vi "_script_uid_display.vi"(9 "Show uid? (F)":bool, 10 "uids":string[](array[string]), 11 "defaults":cluster{"uid":string, "name":string}[](array[cluster])) -> (3 "display":string[](array[string]))   [LabVIEW 2019, in "Script.lvlib"]
doc: "Displays the shortcut with or without the unique identifier formatted as <short name> | <vi>:<arg>.\n\nExample: \"Connect Pane | support\\Builtins.vi:c\"\n\nCreated by: Ryan Pacini"
uses:
  Script.lvlib
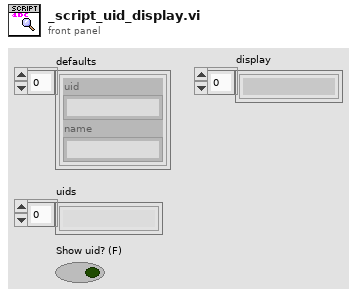
[diagram p1: front panel]
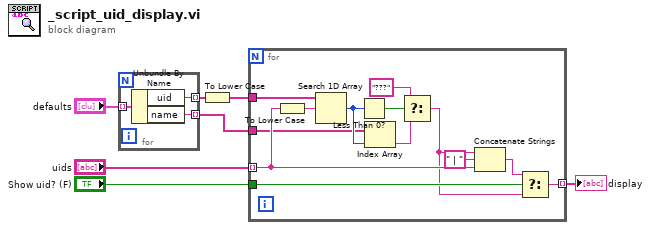
[diagram p0: block diagram]
diagram:
  n1 = for {
    tunnel: "defaults" -> [w10] mode=indexing
    tunnel: [w9] -> w6 mode=indexing
    tunnel: [w8] -> w1 mode=indexing
    n2 = Unbundle By Name(w10) -> ("uid"=w9:string, "name"=w8:string)
  }
  n3 = To Lower Case(string=w6) -> (all lower case string=w5:string[])
  n4 = for {
    tunnel: w5 -> [w23]
    tunnel: "uids" -> [w19] mode=indexing
    tunnel: "Show uid? (F)" -> [w17]
    tunnel: [w14] -> w2 mode=indexing
    tunnel: w1 -> [w12]
    n5 = To Lower Case(string=w19) -> (all lower case string=w22:string)
    n6 = Search 1D Array(1D array=w23, element=w22) -> (index of element=w13:i32)  [unwired: 1 in]
    n7 = Less Than 0?(x=w13) -> (x < 0?=w21:bool)
    n8 = Index Array(array=w12, index=w13) -> (element=w11:string)
    n9 = Select(t="???", s=w21, f=w11) -> (s? t:f=w16:string)
    n10 = Concatenate Strings(w16, " | " ("string"), w19) -> (w18:string)
    n11 = Select(t=w18, s=w17, f=w16) -> (s? t:f=w14:string)
  }
  "display" <- w2
